vi "Key Down.vi"(7 "VKey":T1, 8 "error in":errorcluster, 9 "run":refnum<vi>, 10 "spectrum number":refnum<vi>, 11 "user event \nqueue reference in":refnum<queue>) -> (0 "error out":errorcluster, 3 "user event\nqueue reference out":refnum<queue>)   [LabVIEW 2011]
uses:
  <vilib>/event_ctls.llb/eventvkey.ctl
  Controls/User Event Control.ctl
  Controls/User Event Action.ctl
  Controls/User Interface Action.ctl
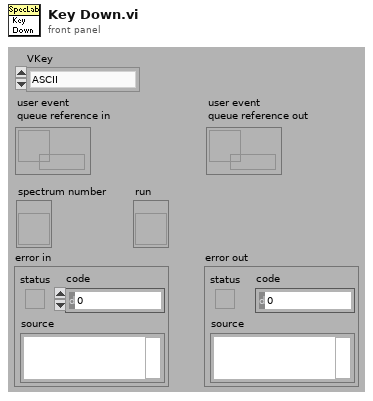
[diagram p1: front panel]
types:
  T1 = typedef "eventvkey.ctl" = enum16{"ASCII", "Enter", "Return", "Shift", "Ctrl", "Alt", "Cmd", "Opt", "Caps", "NumLock", "Clear", "Break", "Up", "Down", "Left", "Right", "Insert", "Delete", "Home", "End", "PageUp", "PageDown", "Escape", "Help", "Pause", "ScrollLock", "F1", "F2", "F3", "F4", "F5", "F6", "F7", "F8", "F9", "F10", "F11", "F12", "F13", "F14", "F15", "F16", "F17", "F18", "F19", "F20", "F21", "F22", "F23", "F24", "Play", "VolumeUp", "VolumeDown", "Mute", "Two Byte Char"}
  T2 = typedef "User Event Control.ctl" = cluster{"action":T3, "data":variant}
  T3 = typedef "User Event Action.ctl" = enum16{"Program Initialization", "Device Connections", "Device Settings", "Options", "DAQ Init", "PID Sample Test", "PID with PS Challenge", "PID with MFC Challenge", "Multimeter Sample Test", "Multimeter with MFC Challenge", "DAQ Stop", "Open Data File", "View Data File", "Change Display Mode", "Load INL PID Run Data", "Load Baseline-Mocon PID Data", "Load Multimeter Data", "Set Channel Sample", "Key Down", "Add Spectrum to Plot", "Add History to Plot", "Export History to Excel", "Clear Plots", "Save Plot", "Save Spectral Variable", "History Cursor Release", "Analysis Plot Cursor Release", "Program Deinitialization"}
  T4 = typedef "User Interface Action.ctl" = enum16{"Initialize", "Data Acquisition Disable", "Data View Disable", "Sample Set", "Sample Set 2D Data", "Sample Set x0 & dx", "Sample Add", "Sample Set Cursor", "Sample Set Offset & Multiplier", "Sample Set Axis Labels", "Sample Parameters Disabled", "Sample Parameters Update", "Run Update", "Run Set Offset & Multiplier", "Run Set Axis Labels", "Run Set Cursor", "Run Set Disabled", "Run Parameters Update", "Run Parameters Disabled", "Run Number Set", "Run Number Set Range", "Run Number Set Disabled", "Sample Number Set", "Sample Number Set Range", "Notes Set Value", "Update Plot", "Set Plot Parameters", "Update Concentration Plot", "Time Set", "Clear DAQ Display", "Clear Analysis Display", "Status Bar Set", "Progress Bar Set", "Display Mode Set", "Experiment Type Set", "Analysis Plot Average Set", "Stop"}
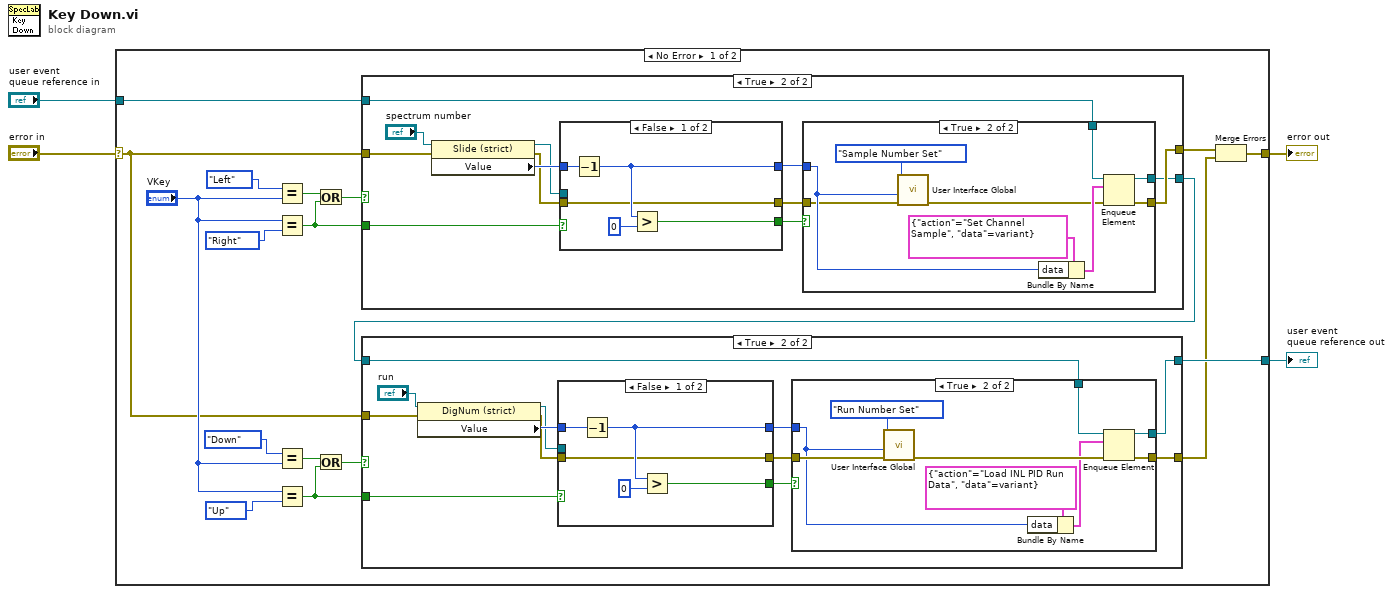
[diagram p0: block diagram]
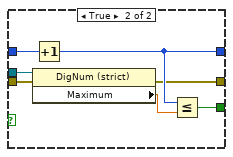
[diagram p4: hidden frame]
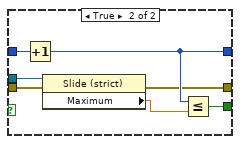
[diagram p6: hidden frame]
diagram:
  n1 = case shown="No Error" "error in" {
    selector: "error in" -> [w11 w98]
    tunnel: [w5 w98] -> w4
    tunnel: "user event \nqueue reference in" -> [w10 w97]
    tunnel: [w8 w97] -> w1
    frame No Error {
      n2 = Equal?(x=eventvkey."Left" ("VKey"), y="VKey") -> (x = y?=w20:bool)
      n3 = Equal?(x="VKey", y=eventvkey."Right" ("VKey")) -> (x = y?=w22:bool)
      n4 = Equal?(x=eventvkey."Down", y="VKey") -> (x = y?=w14:bool)
      n5 = Equal?(x="VKey", y=eventvkey."Up") -> (x = y?=w12:bool)
      n6 = Or(x=w20, y=w22) -> (x .or. y?=w21:bool)
      n7 = Or(x=w14, y=w12) -> (x .or. y?=w13:bool)
      n8 = case shown="True" w21 {
        tunnel: w22 -> [_ w73]
        tunnel: w11 -> [w61 w66]
        tunnel: [w61 w70] -> w6
        tunnel: [w60 w67] -> w9
        tunnel: w10 -> [w60 w62]
        frame False {
        }
        frame True {
          n9 = property class="Slide (strict)"(reference="spectrum number", error in=w66) -> (reference out=w68:refnum<vi>, error out=w65:errorcluster, "Value"=w72:u32)
          n10 = case shown="False" w73 {
            tunnel: w72 -> [w78 w85]
            tunnel: [w77 w83] -> w71
            tunnel: [w75 w82] -> w69
            tunnel: w68 -> [_ w81]
            tunnel: w65 -> [w74 w80]
            tunnel: [w74 w79] -> w64
            frame False {
              n11 = Decrement(x=w78) -> (x-1=w77:u32)
              n12 = Greater?(x=w77, y=0) -> (0:w75:bool)
            }
            frame True {
              n13 = Increment(x=w85) -> (x+1=w83:u32)
              n14 = property on="Property Node" class="Slide (strict)"(reference=w81, error in=w80) -> (error out=w79:errorcluster, "Maximum"=w84:dbl)  [unwired: 1 out]
              n15 = Less Or Equal?(x=w83, y=w84) -> (x <= y?=w82:bool)
            }
          }
          n16 = case shown="True" w69 {
            tunnel: w71 -> [_ w93]
            tunnel: [w86 w95] -> w70
            tunnel: w62 -> [w87 w91]
            tunnel: [w87 w90] -> w67
            tunnel: w64 -> [w86 w89]
            frame False {
            }
            frame True {
              n17 = call "User Interface Global.vi"("error in"=w89, "data1"=w93, "action"=User_Interface_Action."Sample Number Set") -> ("error out"=w88:errorcluster)  [unwired: 8 in]
              n18 = Bundle By Name(cluster=T2 {"action"=enum."Set Channel Sample", "data"=variant} ("element"), "data"=w93) -> (w92:T2)
              n19 = Enqueue Element(queue=w91, element=w92, error in (no error)=w88) -> (queue out=w90:refnum<queue>, error out=w95:errorcluster)  [unwired: 1 in, 1 out]
            }
          }
        }
      }
      n20 = case shown="True" w13 {
        tunnel: w12 -> [_ w36]
        tunnel: w11 -> [w23 w31]
        tunnel: w9 -> [w24 w27]
        tunnel: [w24 w26] -> w8
        tunnel: [w23 w25] -> w7
        frame False {
        }
        frame True {
          n21 = property class="DigNum (strict)"(reference="run", error in=w31) -> (reference out=w34:refnum<vi>, error out=w29:errorcluster, "Value"=w35:u16)
          n22 = case shown="False" w36 {
            tunnel: w35 -> [w51 w59]
            tunnel: w34 -> [_ w58]
            tunnel: [w50 w56] -> w32
            tunnel: [w49 w55] -> w33
            tunnel: w29 -> [w48 w54]
            tunnel: [w48 w53] -> w28
            frame False {
              n23 = Decrement(x=w51) -> (x-1=w50:u16)
              n24 = Greater?(x=w50, y=0) -> (0:w49:bool)
            }
            frame True {
              n25 = property class="DigNum (strict)"(reference=w58, error in=w54) -> (error out=w53:errorcluster, "Maximum"=w57:dbl)  [unwired: 1 out]
              n26 = Increment(x=w59) -> (x+1=w56:u16)
              n27 = Less Or Equal?(x=w56, y=w57) -> (x <= y?=w55:bool)
            }
          }
          n28 = case shown="True" w33 {
            tunnel: w32 -> [_ w41]
            tunnel: w28 -> [w38 w46]
            tunnel: w27 -> [w37 w44]
            tunnel: [w37 w40] -> w26
            tunnel: [w38 w39] -> w25
            frame False {
            }
            frame True {
              n29 = call "User Interface Global.vi"("error in"=w46, "data1"=w41, "action"=User_Interface_Action."Run Number Set") -> ("error out"=w45:errorcluster)  [unwired: 8 in]
              n30 = Bundle By Name(cluster=T2 {"action"=enum."Load INL PID Run Data", "data"=variant} ("element"), "data"=w41) -> (w42:T2)
              n31 = Enqueue Element(queue=w44, element=w42, error in (no error)=w45) -> (queue out=w40:refnum<queue>, error out=w39:errorcluster)  [unwired: 1 in, 1 out]
            }
          }
        }
      }
      n32 = Merge Errors(w6, w7) -> (w5:errorcluster)
    }
    frame Error {
    }
  }
  "error out" <- w4
  "user event\nqueue reference out" <- w1
